vi "Frame.vi"(8 "error in (no error)":errorcluster, 9 "Frame Instruction":T1, 10 "PN sequence order (9)":i32=9, 11 "array":i8[](array[numeric])) -> (0 "error out":errorcluster, 3 "appended array":i8[](array[numeric]))   [LabVIEW 2014]
uses:
  <vilib>/addons/Modulation/Digital/General/MT Generate Bits (Galois, PN Order).vi
  <vilib>/addons/Modulation/Digital/Support/Common/Validators/mod_Generate Bits Validate.vi
  <vilib>/addons/Modulation/Analog/support/mod_Set Error Source.vi
  <vilib>/addons/Modulation/Digital/General/subVIs/mod_Generate Bits PN Sequence.vi
  <vilib>/addons/Modulation/niDMT.lvlib
panel:
  out "array 2":i8[](array[numeric])
  out "number":u32
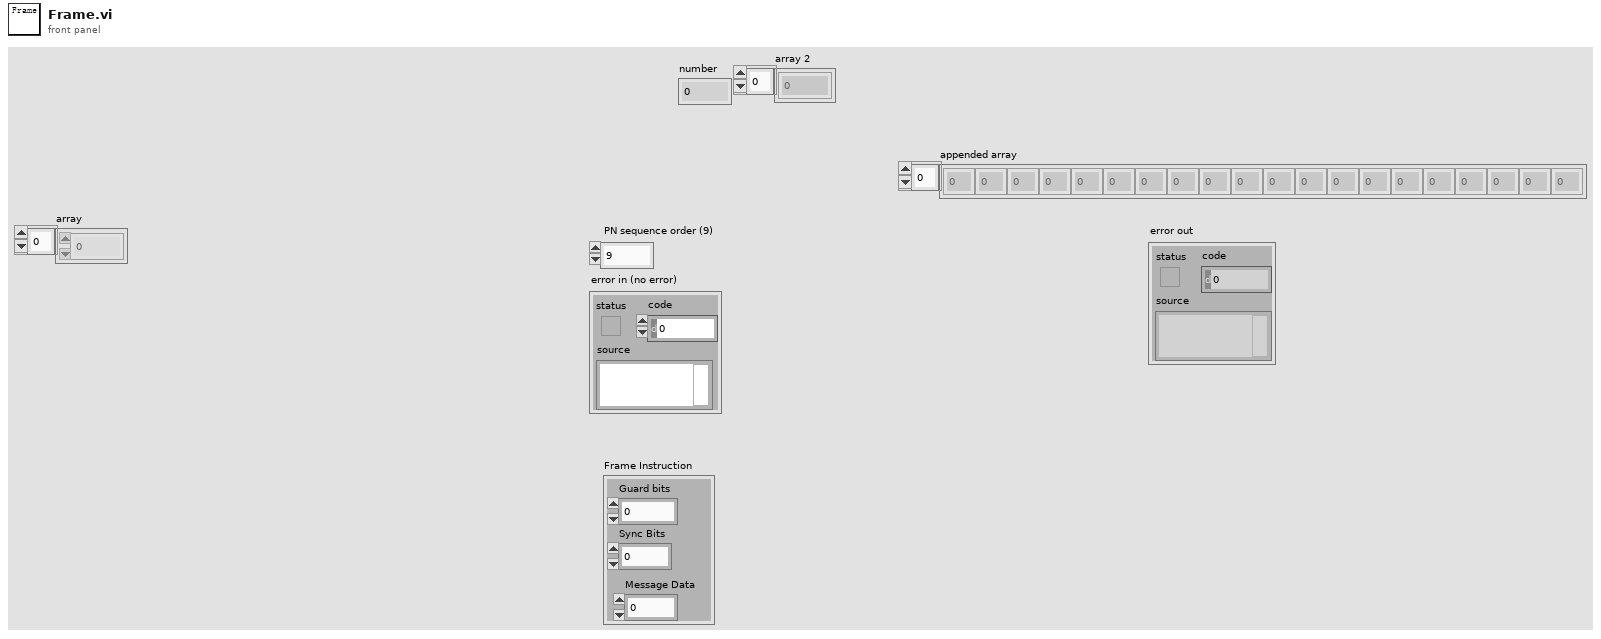
[diagram p1: front panel]
types:
  T1 = cluster{"Guard bits":dbl, "Sync Bits":dbl, "Message Data":dbl}
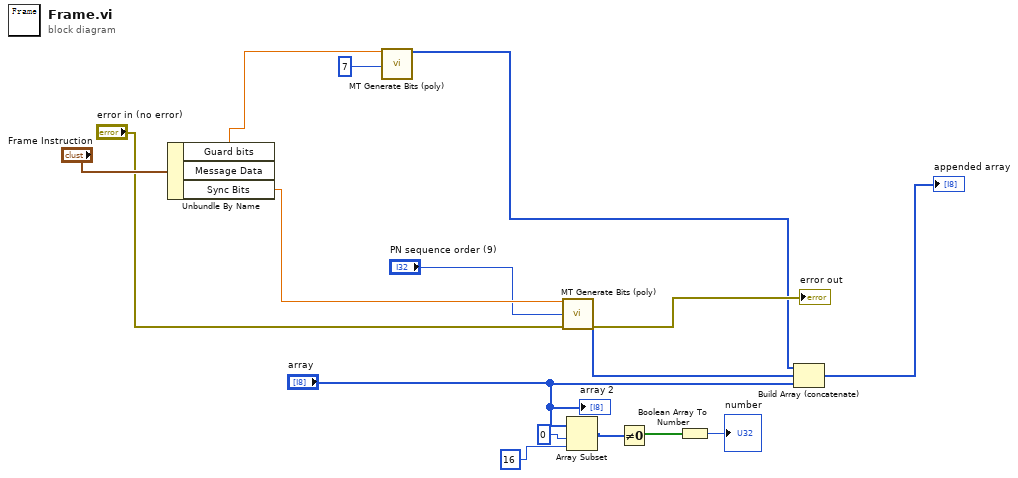
[diagram p0: block diagram]
diagram:
  n1 = Unbundle By Name("Frame Instruction") -> ("Guard bits"=w8:dbl, "Sync Bits"=w13:dbl)  [unwired: 1 out]
  n2 = call-poly <vilib>:"MT Generate Bits (poly).vi"("total bits (128)"=w8, "PN sequence order (9)"=7) -> ("output bit stream"=w7:i8[])  [unwired: 11 in, 2 out]
  n3 = call-poly <vilib>:"MT Generate Bits (poly).vi"("total bits (128)"=w13, "PN sequence order (9)"="PN sequence order (9)", "error in (no error)"="error in (no error)") -> ("output bit stream"=w14:i8[], "error out"=→"error out":errorcluster)  [unwired: 10 in, 1 out]
  n4 = Array Subset(array="array", index=0, length=16) -> (w4:i8[])
  n5 = Not Equal To 0?(x=w4) -> (x != 0?=w3:bool[])
  n6 = Boolean Array To Number(Boolean array=w3) -> (number=→"number":u32)
  n7 = Build Array (concatenate) "Build Array"(w7, w14, "array") -> (→"appended array":i8[])
  "array 2" <- "array"
